vi "Read from Hardware.vi"(8 "error in":errorcluster, 10 "values":dbl[](array[numeric]), 11 "rx execution unit":refnum<class "Rx Execution Unit.lvclass">) -> (0 "error out":errorcluster, 2 "values out":dbl[](array[numeric]), 3 "rx execution unit out":refnum<class "Rx Execution Unit.lvclass">)   [LabVIEW 2020, in "AIM MIL-STD-1553 Engine.lvlib" / "Implementation.lvlib" / "Rx Execution Unit.lvclass"]
uses:
  Rx Execution Unit.lvclass
  Execution Unit/Execution Unit.lvclass/Execution Unit.ctl
  Rx Execution Unit.lvclass/Rx Execution Unit.ctl
  Read Received Messages.vi
  Hardware API/AIM MIL-STD-1553 Hardware API.lvlib
  Execution Unit/Execution Unit.lvclass
  C:/dev/git/niveristand-aim-milStd1553-custom-device/Source/Custom Device Support/Engine/Implementation/Execution Unit/Execution Unit.lvclass
  C:/dev/git/niveristand-aim-milStd1553-custom-device/Source/Custom Device Support/Engine/Interfaces/Execution Unit/Execution Unit.lvclass
  C:/dev/git/niveristand-aim-milStd1553-custom-device/Source/Custom Device Support/Engine/Implementation/Rx Execution Unit/Rx Execution Unit.lvclass
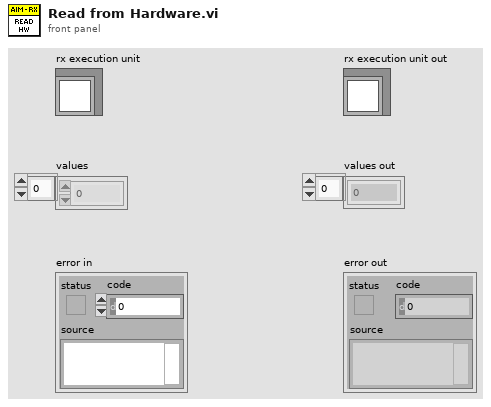
[diagram p1: front panel]
types:
  T1 = typedef "AIM MIL-STD-1553 Hardware API.lvlib/Module Reference.ctl" = u32
  T2 = typedef "AIM MIL-STD-1553 Engine.lvlib/Custom Device.lvlib/Compiled Message.ctl" = cluster{"Message Section Handle":T3, "First Parameter Index":i32, "Parameter Channel Handles":T3[], "Direction":T4, "Parameters":T5[], "Receiving RT Address":u8, "Receiving RT Sub-address":u8, "Transmitting RT Address":u8, "Transmitting RT Sub-address":u8, "Word Count":u8, "Buffer Type":enum16{"unknown", "BC Message Buffer", "RT Message Buffer"}, "Buffer ID":u16, "Terminal Type":enum16{"Bus Controller", "Remote Terminal"}, "Timestamp Enabled":bool, "Timestamp Channel Handle":T3}
  T3 = typedef "Custom Device API.lvlib/Custom Device Item Ref.ctl" = u64
  T4 = typedef "Direction.ctl" = enum16{"Rx", "Tx"}
  T5 = typedef "Parameter Definition.ctl" = cluster{"start index":i32, "size (bits)":i32, "encoding":enum16{"BNR", "BCD", "Discrete"}, "signed":bool, "multiplier":dbl, "offset":dbl}
  T6 = enum16{"unknown", "BC Message Buffer", "RT Message Buffer"}
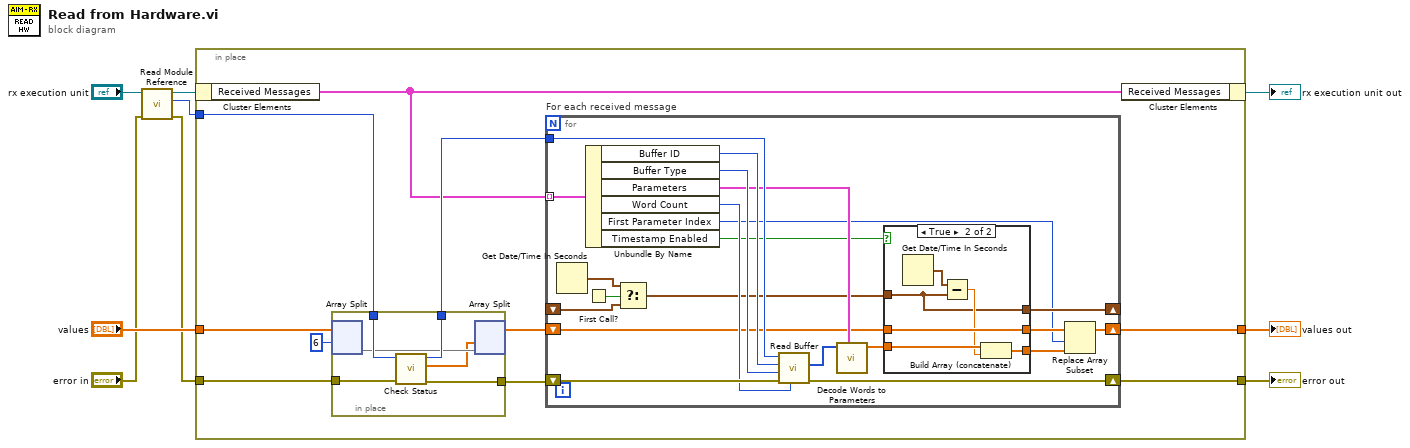
[diagram p0: block diagram]
diagram:
  n1 = call "Read Module Reference.vi"("error in"="error in", "execution unit"="rx execution unit") -> ("error out"=w1:errorcluster, "module reference"=w4:T1, "execution unit out"=w5:refnum<class "Rx Execution Unit.lvclass">)  [unwired: 7 in]
  n2 = in-place {
    in-place-border: [w19] -> w9
    in-place-border: w1 -> [w18]
    in-place-border: "values" -> [w12]
    in-place-border: [w15] -> w7
    in-place-border: w4 -> [w14]
    n3 = in-place-cluster #1(w5) -> ("Received Messages"=w13:T2[])
    n4 = in-place {
      in-place-border: w18 -> [w25]
      in-place-border: [w24] -> w17
      in-place-border: [w23] -> w16
      in-place-border: w14 -> [w22]
      n5 = in-place-split #2(w12, 6) -> (w21:dbl[])  [unwired: 1 out]
      n6 = call "Check Status.vi"("error in"=w25, "module handle"=w22) -> ("error out"=w24:errorcluster, "status values"=w20:dbl[], "module handle out"=w23:u32)  [unwired: 7 in]
      n7 = in-place-split #2(w20, w21) -> (w10:dbl[])  [unwired: 1 out]
    }
    n8 = for "For each received message" {
      tunnel: w13 -> [w46] mode=indexing
      tunnel: w16 -> [w45]
      shift-right: [w39] -> w19
      shift-left: w17 -> [w42]
      shift-right: [w40] -> w15
      shift-left: w10 -> [w32]
      shift-right: [w27] -> _
      shift-left: _ -> [w29]
      n9 = Get Date/Time In Seconds() -> (seconds since 1Jan1904=w30:timestamp)
      n10 = First Call?() -> (First Call?: T/F=w31:bool)
      n11 = Unbundle By Name(w46) -> ("Buffer ID"=w44:u16, "Buffer Type"=w43:T6, "Parameters"=w41:T5[], "Word Count"=w38:u8, "First Parameter Index"=w26:i32, "Timestamp Enabled"=w34:bool)
      n12 = Select(t=w30, s=w31, f=w29) -> (s? t:f=w28:timestamp)
      n13 = call "Read Buffer.vi"("data length (32)"=w38, "error in"=w42, "buffer type"=w43, "buffer id"=w44, "module handle"=w45) -> ("error out"=w39:errorcluster, "data array out"=w37:u16[])  [unwired: 3 in, 2 out]
      n14 = call "Decode Words to Parameters.vi"("parameters"=w41, "data words"=w37) -> ("Values"=w36:dbl[])  [unwired: 9 in]
      n15 = case shown="True" w34 {
        tunnel: w36 -> [w48 w55]
        tunnel: [w48 w54] -> w35
        tunnel: [w49 w53] -> w33
        tunnel: w32 -> [w49 w53]
        tunnel: w28 -> [w47 w50]
        tunnel: [w47 w50] -> w27
        frame False {
        }
        frame True {
          n16 = Get Date/Time In Seconds() -> (seconds since 1Jan1904=w52:timestamp)
          n17 = Subtract(x=w52, y=w50) -> (x-y=w51:dbl)
          n18 = Build Array (concatenate)(w55, w51) -> (w54:dbl[])
        }
      }
      n19 = Replace Array Subset(array=w33, new element=w35, index=w26) -> (w40:dbl[])
    }
    n20 = in-place-cluster #1("Received Messages"=w13) -> (→"rx execution unit out":refnum<class "Rx Execution Unit.lvclass">)
  }
  "error out" <- w9
  "values out" <- w7
